vi "RenderClear.vi"(8 "No Error":errorcluster, 11 "renderer [SDL_Renderer *]":i64) -> (0 "error out":errorcluster)   [LabVIEW 2024, in "SDL3.lvlib" / "Render.lvlib"]
uses:
  Render.lvlib
  Error/Error.lvlib
  Lib/SDL3-32.dll
panel:
  # "https://wiki.libsdl.org/SDL3/SDL_RenderClear"
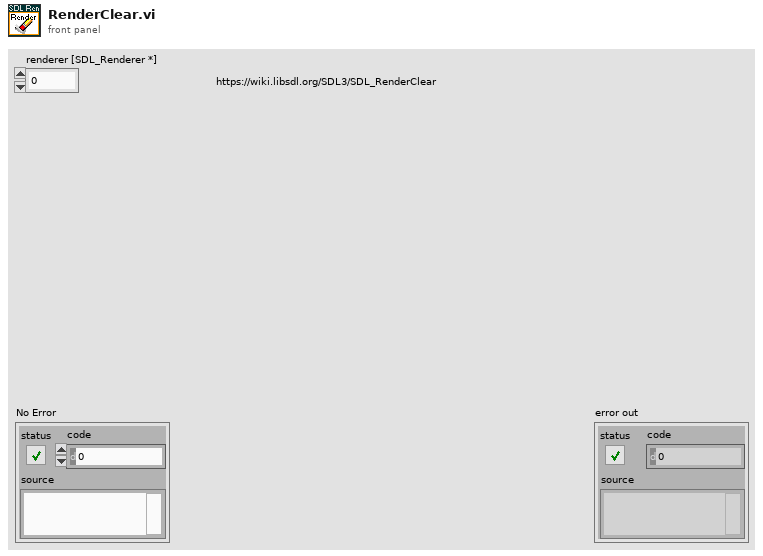
[diagram p1: front panel]
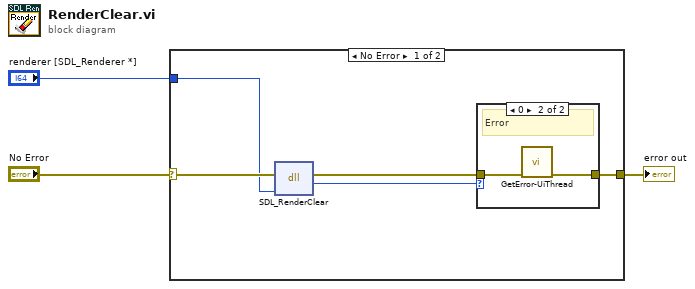
[diagram p0: block diagram]
diagram:
  n1 = case shown="No Error" "No Error" {
    selector: "No Error" -> [w8 w12]
    tunnel: [w6 w12] -> w2
    tunnel: "renderer [SDL_Renderer *]" -> [w4 _]
    frame No Error {
      n2 = dll-call lib="C:/Users/Thomas/Documents/Projects/LV-SDL3/Lib/SDL3-*.*" fn="SDL_RenderClear"(error in=w8, "renderer"=w4) -> (error out=w7:errorcluster, "return type"=w5:i32)  [unwired: 3 in, 1 out]
      n3 = case shown="0" w5 {
        tunnel: w7 -> [w9 w11]
        tunnel: [w9 w10] -> w6
        frame Default {
          # "Ok"
        }
        frame 0 {
          # "Error"
          n4 = call "GetError-UiThread.vi"("No Error"=w11) -> ("error out"=w10:errorcluster)  [unwired: 10 in]
        }
      }
    }
    frame Error {
    }
  }
  "error out" <- w2
